vi "Message.vi"(8 "error in (no error)":errorcluster, 10 "Message":string, 11 "Event_TextLog in":refnum<class "Event_TextLog.lvclass">) -> (0 "error out":errorcluster, 3 "Event_TextLog out":refnum<class "Event_TextLog.lvclass">)   [LabVIEW 2021, in "Event_TextLog.lvclass"]
uses:
  Event_TextLog.lvclass
  C:/Users/Tim/Documents/GitHub/Event_log/Source/abs_EventLog/abs_EventLog.lvclass
  abs_EventLog/abs_EventLog.lvclass/abs_EventLog.ctl
  Event_TextLog.lvclass/Event_TextLog.ctl
  abs_EventLog/Properties/Read Severity Code.vi
  abs_EventLog/Properties/Read Facility Code.vi
  abs_EventLog/Properties/Read Message Tag.vi
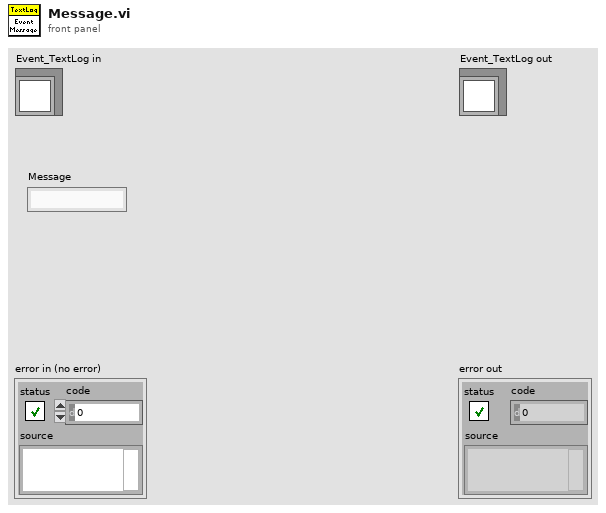
[diagram p1: front panel]
types:
  T1 = typedef "abs_EventLog.lvclass/Severity Code.ctl" = enum16{"emergency", "alert", "critical", "error", "warning", "notice", "info", "debug"}
  T2 = typedef "abs_EventLog.lvclass/Facility Code.ctl" = enum16{"kernel", "user", "mail", "system daemons", "security/authorization", "syslogd", "line printer", "network news", "uucp", "clock daemon", "security/authorization (alternate)", "FTP daemon", "NTP subsystem", "log audit", "log alert", "clock daemon (alternate)", "local use 0", "local use 1", "local use 2", "local use 3", "local use 4", "local use 5", "local use 6", "local use 7"}
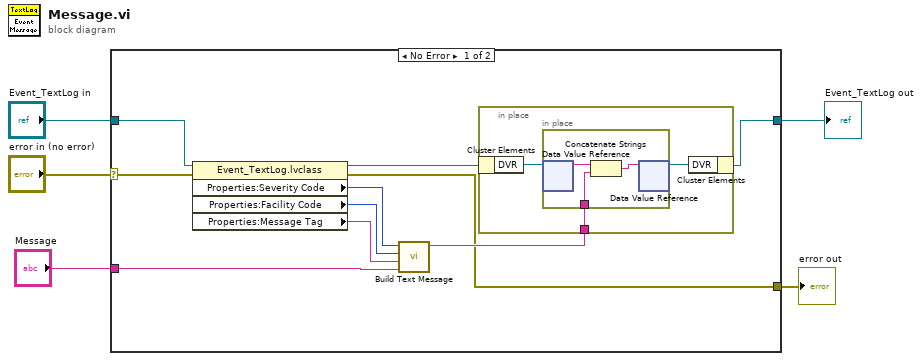
[diagram p0: block diagram]
diagram:
  n1 = case shown="No Error" "error in (no error)" {
    selector: "error in (no error)" -> [w10 w22]
    tunnel: "Message" -> [w15 _]
    tunnel: "Event_TextLog in" -> [w14 w23]
    tunnel: [w8 w23] -> w2
    tunnel: [w6 w22] -> w1
    frame No Error {
      n2 = property class="Event_TextLog.lvclass"(reference=w14, error in=w10) -> (reference out=w9:refnum<class "Event_TextLog.lvclass">, error out=w6:errorcluster, "Properties:Severity Code"=w13:T1, "Properties:Facility Code"=w12:T2, "Properties:Message Tag"=w11:string)
      n3 = call "Build Text Message.vi"("Message Content"=w15, "Message Tag"=w11, "Facility Code"=w12, "Severity Code"=w13) -> ("Syslog Message"=w7:string)  [unwired: 7 in]
      n4 = in-place {
        in-place-border: w7 -> [w16]
        n5 = in-place-cluster #1(w9) -> ("DVR"=w18:refnum<data-value>)
        n6 = in-place {
          in-place-border: w16 -> [w19]
          n7 = in-place-dvr #2(w18) -> (w21:string)  [unwired: 1 out]
          n8 = Concatenate Strings(w21, w19) -> (w20:string)
          n9 = in-place-dvr #2(w20) -> (w17:refnum<data-value>)  [unwired: 1 out]
        }
        n10 = in-place-cluster #1("DVR"=w17) -> (w8:refnum<class "Event_TextLog.lvclass">)
      }
    }
    frame Error {
    }
  }
  "error out" <- w1
  "Event_TextLog out" <- w2
